vi "Calc_rhominus.vi"(10 "Q":dbl[](array[numeric]), 11 "P":dbl[](array[numeric])) -> (3 "rho+":dbl[](array[numeric]))   [LabVIEW 2018]
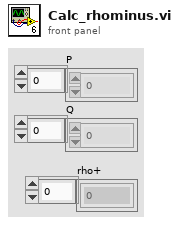
[diagram p1: front panel]
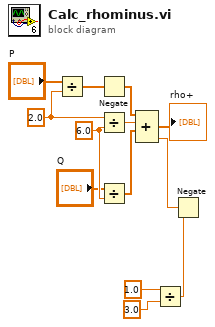
[diagram p0: block diagram]
diagram:
  w11 = 6.0
  w12 = 2.0
  n1 = Divide(x="P", y=w12) -> (x/y=w7:dbl[])
  n2 = Negate(x=w7) -> (-x=w5:dbl[])
  n3 = Divide(x=w12, y=w11) -> (x/y=w9:dbl)
  n4 = Divide(x="Q", y=w11) -> (x/y=w8:dbl[])
  n5 = Divide(x=1.0, y=3.0) -> (x/y=w2:dbl)
  n6 = Negate(x=w2) -> (-x=w1:dbl)
  n7 = Compound Arithmetic op=ADD(w5, w9, w8, w1) -> (→"rho+":dbl[])
